vi "DSF.Engine.Memory.Buffer.Write.1D.I8.vi"(7 "count (-1: all)":i64=-1 format="%d elements", 8 "error in (no error)":errorcluster, 9 "offset (0)":u64 format="%d bytes", 10 "buffer in":i8[](array[numeric]), 11 "Buffer in":refnum<class "DSF.Engine.Memory.Buffer.lvclass">) -> (0 "error out":errorcluster, 1 "offset out":u64 format="%d bytes", 2 "buffer out":i8[](array[numeric]), 3 "Buffer out":refnum<class "DSF.Engine.Memory.Buffer.lvclass">)   [LabVIEW 2017, in "DSF.Engine.lvlib" / "DSF.Engine.Memory.Buffer.lvclass"]
uses:
  DSF.Engine.Memory.Buffer.lvclass
  C:/Git/DSF/dsf core/Built/Windows/Dependencies/Memory Manager.lvlibp/1abvi3w/vi.lib/National Instruments/Memory Manager/Classes/Pointer/Memory.Pointer.lvclass
  Built/PharLap x86/Dependencies/c/Memory Manager.lvlibp/1abvi3w/vi.lib/National Instruments/Memory Manager/Classes/Pointer/Memory.Pointer.Write.1D.I8.vi
  Built/PharLap x86/Dependencies/c/Memory Manager.lvlibp/1abvi3w/vi.lib/National Instruments/Memory Manager/Classes/Pointer/Memory.Pointer.lvclass
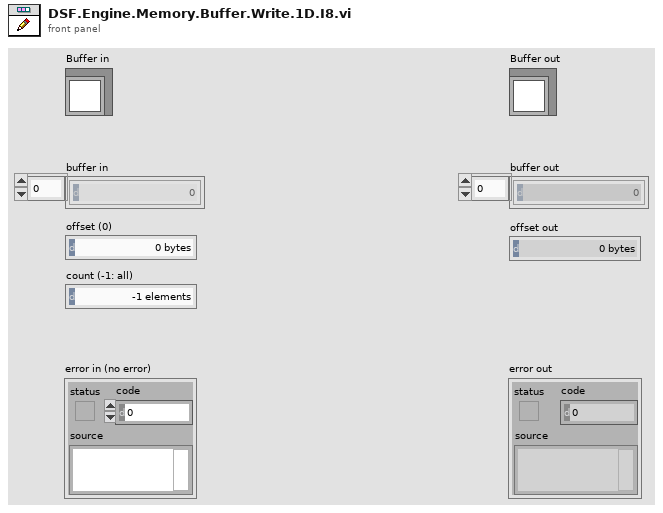
[diagram p1: front panel]
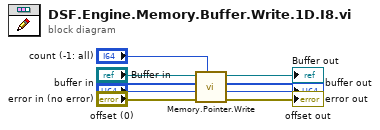
[diagram p0: block diagram]
diagram:
  n1 = call-poly "Memory.Pointer.Write.vi"("count (-1: all)"="count (-1: all)", "error in (no error)"="error in (no error)", "offset (0)"="offset (0)", "buffer in"="buffer in", "Pointer in"="Buffer in") -> ("error out"=→"error out":errorcluster, "offset out"=→"offset out":u64, "buffer out"=→"buffer out":i8[], "Pointer out"=→"Buffer out":refnum<class "DSF.Engine.Memory.Buffer.lvclass">)  [unwired: 3 in]
